vi "ResetAngleWithOffsetFunction.vi"(10 "Offset":dbl[](array[numeric]), 11 "AngleInput":dbl[](array[numeric])) -> (3 "AngleOutput":dbl[](array[numeric]))   [LabVIEW 2018]
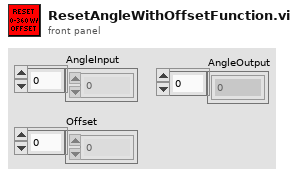
[diagram p1: front panel]
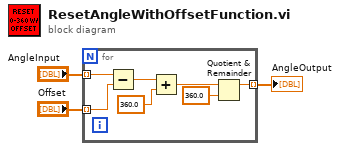
[diagram p0: block diagram]
diagram:
  n1 = for {
    tunnel: "AngleInput" -> [w10] mode=indexing
    tunnel: "Offset" -> [w9] mode=indexing
    tunnel: [w8] -> w1 mode=indexing
    n2 = Subtract(x=w10, y=w9) -> (x-y=w7:dbl)
    n3 = Add(x=w7, y=360.0) -> (x+y=w5:dbl)
    n4 = Quotient & Remainder(x=w5, y=360.0) -> (x-y*floor(x/y)=w8:dbl)  [unwired: 1 out]
  }
  "AngleOutput" <- w1
